vi "read_data (SubVI).vi"(0 "data tasks":T2) -> (1 "output data tasks":T1, 2 "Output data":dbl[][](array[numeric]), 3 "Rescaled data":i16[][](array[numeric]), 4 "sample rate":dbl)   [LabVIEW 2016]
uses:
  <vilib>/DAQmx/read.llb/DAQmx Read (Analog 2D DBL NChan NSamp).vi
  <vilib>/DAQmx/miscellaneous.llb/DAQmx Fill In Error Info.vi
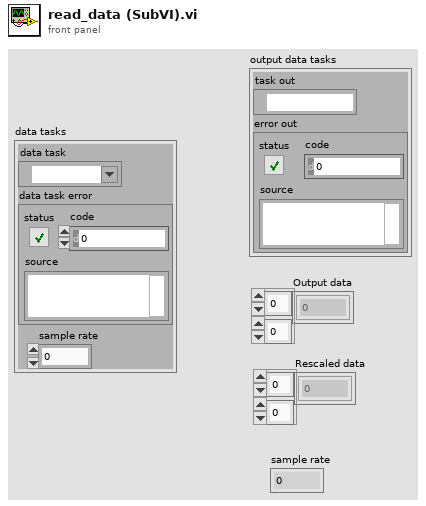
[diagram p1: front panel]
types:
  T1 = cluster{"task out":refnum<k21>, "error out":errorcluster}
  T2 = cluster{"data task":refnum<k21>, "data task error":errorcluster, "sample rate":dbl}
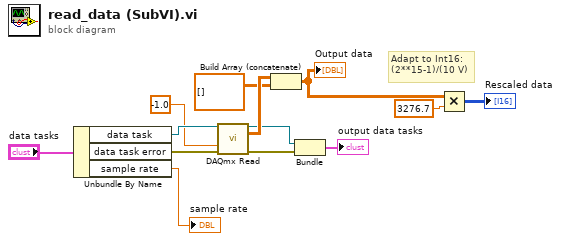
[diagram p0: block diagram]
diagram:
  # "Adapt to Int16: \n(2**15-1)/(10 V)"
  n1 = Unbundle By Name("data tasks") -> ("data task"=w12:refnum<k21>, "data task error"=w11:errorcluster, "sample rate"=→"sample rate":dbl)
  n2 = call-poly <vilib>:"DAQmx Read.vi"("task/channels in"=w12, "timeout"=-1.0, "error in"=w11) -> ("task out"=w6:refnum<k21>, "data"=w9:dbl[][], "error out"=w5:errorcluster)  [unwired: 10 in]
  n3 = Build Array (concatenate)(w9, dbl[][] [] ("array")) -> (w7:dbl[][])
  "Output data" <- w7
  n4 = Bundle("task out"=w6, "error out"=w5) -> (→"output data tasks":T1)  [unwired: 1 in]
  n5 = Multiply(x=w7, y=3276.7) -> (x*y=→"Rescaled data":i16[][])
